vi "CurrencyUpdate.vi"(8 "error in (no error)":errorcluster, 11 "Coins in":refnum<class "Coins.lvclass">) -> (0 "error out":errorcluster, 3 "Coins out":refnum<class "Coins.lvclass">)   [LabVIEW 2020, in "Coins.lvlib" / "Coins.lvclass"]
uses:
  Coins.lvclass
  Coins.lvclass/Coins.ctl
  Read Currency.vi
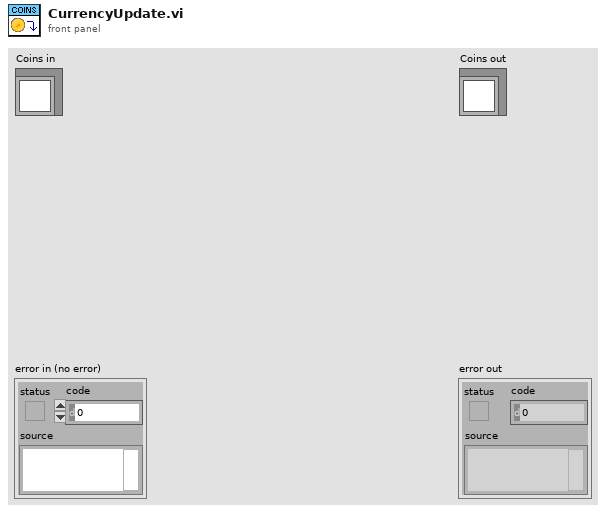
[diagram p1: front panel]
types:
  T1 = typedef "Currency Enum.ctl" = enum16{"USD", "MXN", "EUR"}
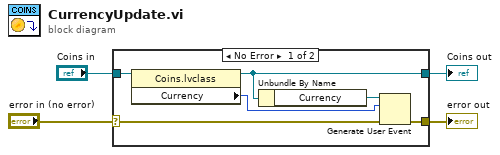
[diagram p0: block diagram]
diagram:
  n1 = case shown="No Error" "error in (no error)" {
    selector: "error in (no error)" -> [w10 w12]
    tunnel: [w9 w12] -> w3
    tunnel: [w6 w11] -> w1
    tunnel: "Coins in" -> [w8 w11]
    frame No Error {
      n2 = property class="Coins.lvclass"(reference=w8) -> (reference out=w6:refnum<class "Coins.lvclass">, "Currency"=w5:T1)  [unwired: 1 in, 1 out]
      n3 = Unbundle By Name(w6) -> ("Currency"=w7:refnum<user-event>)
      n4 = Generate User Event(user event=w7, event data cluster=w5, error in=w10) -> (error out=w9:errorcluster)  [unwired: 1 in, 1 out]
    }
    frame Error {
    }
  }
  "error out" <- w3
  "Coins out" <- w1
